vi "NI VeriStand - Get Item Reference by Path.vi"(8 "error in (no error)":errorcluster, 10 "Root Ref":T1=18446744073709551615 format="%.0x", 11 "Item Path in":string) -> (0 "error out":errorcluster, 2 "Item Ref":T1 format="%.0x", 3 "Item Path out":string, 4 "Found":bool)   [LabVIEW 2020, in "Custom Device Offline API.lvlib"]
uses:
  <vilib>/NI VeriStand/Custom Device Offline API/Custom Device Offline API.lvlib
  <vilib>/NI VeriStand/Custom Device API/Custom Device Item Ref.ctl
  NationalInstruments.VeriStand.SystemDefinitionAPI
  <vilib>/NI VeriStand/Custom Device API/Custom Device API.lvlib
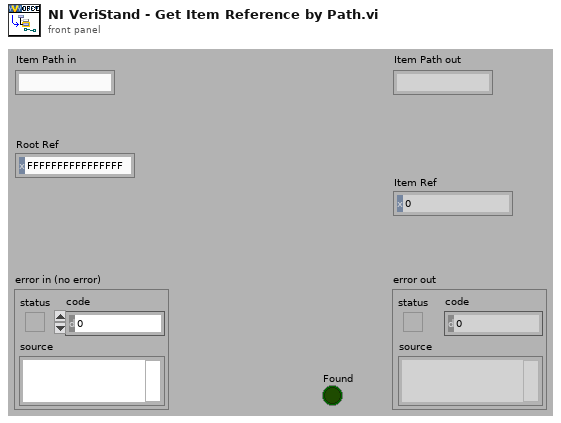
[diagram p1: front panel]
types:
  T1 = typedef "Custom Device API.lvlib/Custom Device Item Ref.ctl" = u64
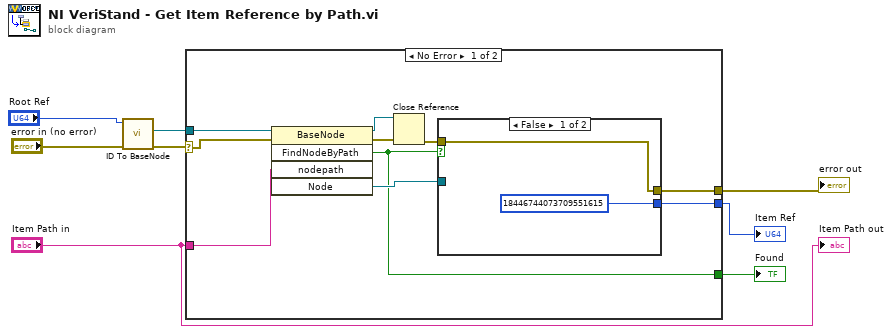
[diagram p0: block diagram]
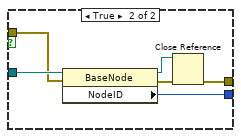
[diagram p2: hidden frame]
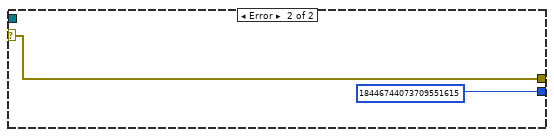
[diagram p3: hidden frame]
diagram:
  n1 = call <vilib>:"ID To BaseNode.vi"("error in (no error)"="error in (no error)", "ID in"="Root Ref") -> ("error out"=w7:errorcluster, "BaseNode"=w5:refnum<k24>)  [unwired: 7 in, 1 out]
  n2 = case shown="No Error" w7 {
    selector: w7 -> [w17 w28]
    tunnel: w5 -> [w18 _]
    tunnel: "Item Path in" -> [w16 _]
    tunnel: [w11 T1 18446744073709551615 ("Item Ref")] -> w3
    tunnel: [w10 w28] -> w2
    tunnel: [w9 _] -> w1
    frame No Error {
      n3 = invoke class="BaseNode" method="FindNodeByPath"(reference=w18, error in=w17, "nodepath"=w16) -> (reference out=w14:refnum<k24>, error out=w15:errorcluster, "FindNodeByPath"=w9:bool, "Node"=w13:refnum<k24>)  [unwired: 2 in, 1 out]
      n4 = Close Reference(reference=w14, error in (no error)=w15) -> (error out=w12:errorcluster)
      n5 = case shown="False" w9 {
        tunnel: w13 -> [_ w26]
        tunnel: w12 -> [w19 w25]
        tunnel: [T1 18446744073709551615 ("Item Ref") w22] -> w11
        tunnel: [w19 w21] -> w10
        frame False {
        }
        frame True {
          n6 = property class="BaseNode"(reference=w26, error in=w25) -> (reference out=w23:refnum<k24>, error out=w24:errorcluster, "NodeID"=w22:u64)
          n7 = Close Reference(reference=w23, error in (no error)=w24) -> (error out=w21:errorcluster)
        }
      }
    }
    frame Error {
    }
  }
  "error out" <- w2
  "Found" <- w1
  "Item Ref" <- w3
  "Item Path out" <- "Item Path in"
